vi "PH_Beamline_Common.set Linear Stage.vi"(1 "Alignment (vertical)":T1=enum."vertical", 2 "CtlRef":refnum<vi>, 4 "GUI Instance does not exist or here?":bool, 5 "error in (no error)":errorcluster) -> (19 "error out":errorcluster)   [LabVIEW 2014, in "PH_Beamline_Common.lvlib"]
uses:
  PH_Beamline_Common.lvlib
  PH_Common/Picture/PH_Picture.Alignment.ctl
  PH_Common/PH_Common.lvlib
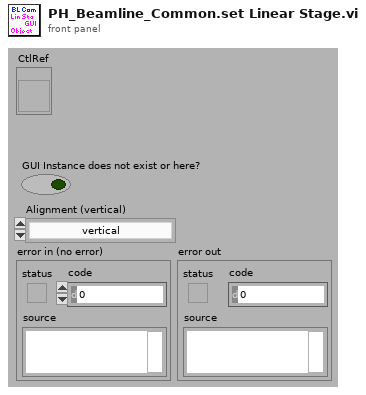
[diagram p1: front panel]
types:
  T1 = typedef "PH_Common.lvlib/PH_Picture.Alignment.ctl" = enum16{"neutral", "left", "right", "up", "down", "vertical", "horizontal", "left down to right up", "left up to right down"}
  T2 = cluster{"left":i16, "top":i16, "right":i16, "bottom":i16}
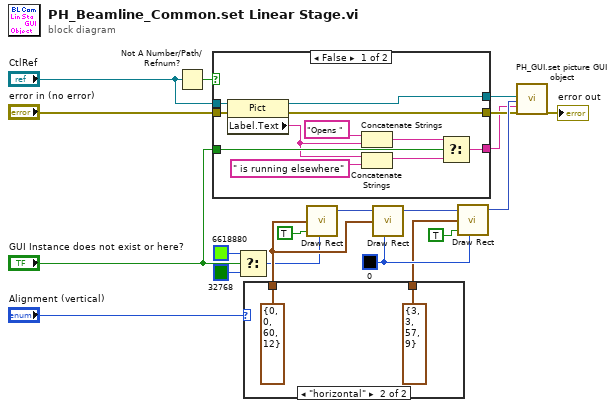
[diagram p0: block diagram]
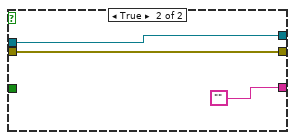
[diagram p2: hidden frame]
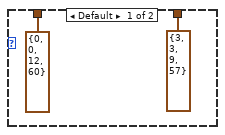
[diagram p3: hidden frame]
diagram:
  w3 = u32 0
  n1 = Not A Number/Path/Refnum?(number/path/refnum="CtlRef") -> (NaN/Path/Refnum?=w14:bool)
  n2 = case shown="False" w14 {
    tunnel: "CtlRef" -> [w30 w34]
    tunnel: "error in (no error)" -> [w29 w33]
    tunnel: [w28 w34] -> w10
    tunnel: [w27 w33] -> w12
    tunnel: [w23 ""] -> w9
    tunnel: "GUI Instance does not exist or here?" -> [w22 _]
    frame False {
      n3 = property class="Pict"(reference=w30, error in=w29) -> (reference out=w28:refnum<vi>, error out=w27:errorcluster, "Label.Text"=w21:string)
      n4 = Concatenate Strings("Opens " ("string"), w21) -> (w24:string)
      n5 = Concatenate Strings(w21, " is running elsewhere" ("string")) -> (w25:string)
      n6 = Select(t=w24, s=w22, f=w25) -> (s? t:f=w23:string)
    }
    frame True {
    }
  }
  n7 = Select(t=u32 6618880, s="GUI Instance does not exist or here?", f=u32 32768 ("Color Box")) -> (s? t:f=w4:u32)
  n8 = case shown="\"horizontal\"" "Alignment (vertical)" {
    tunnel: [T2 {"left"=3, "top"=3, "right"=9, "bottom"=57} ("rect") T2 {"left"=3, "top"=3, "right"=57, "bottom"=9} ("rect")] -> w1
    tunnel: [T2 {"left"=0, "top"=0, "right"=12, "bottom"=60} ("rect") T2 {"left"=0, "top"=0, "right"=60, "bottom"=12} ("rect")] -> w16
    frame Default {
    }
    frame "horizontal" {
    }
  }
  n9 = call <vilib>:"Draw Rect.vi"("rect"=w16, "fill?(F)"=TRUE, "color(black)"=w4) -> ("new picture"=w17:picture)  [unwired: 6 in]
  n10 = call <vilib>:"Draw Rect.vi"("picture"=w17, "rect"=w16, "color(black)"=w3) -> ("new picture"=w5:picture)  [unwired: 6 in]
  n11 = call <vilib>:"Draw Rect.vi"("picture"=w5, "rect"=w1, "fill?(F)"=TRUE, "color(black)"=w3) -> ("new picture"=w18:picture)  [unwired: 5 in]
  n12 = call "PH_GUI.set picture GUI object.vi"("CtlRef"=w10, "Picture"=w18, "Tip Strip (\"\")"=w9, "error in (no error)"=w12) -> ("error out"=→"error out":errorcluster)  [unwired: 15 in]
